vi "探头启用设置.vi"() -> ()   [LabVIEW 2016, in "斯坦道多参数.lvlib"]
uses:
  <vilib>/Utility/miscctls.llb/LVPointTypeDef.ctl
panel:
  in  "藻密度单位":enum16{"cells/mL", "cells/L"}(ring)
  in  "叶绿素a单位":enum16{"μg/L", "mg/L"}(ring)
  in  "关闭":bool
  in  "水温通道":u16(ring)=1 items=["pH", "DO", "浊度", "电导率", "叶绿素a", "藻密度"]
  in  "DO2探头选择":u16(ring)=1 items=["YL型", "MQ型", "NAQ型"]
  in  "DO2启用":bool
  in  "COD探头选择":u16(ring)=1 items=["YL型", "MQ型", "NAQ型"]
  in  "COD启用":bool
  in  "pH":bool
  in  "DO":bool
  in  "Turb":bool
  in  "Cond":bool
  in  "Temp":bool
  in  "叶绿素a启用":bool
  in  "藻密度":bool
  in  "pH探头选择":u16(ring) items=["YL型", "MQ型", "NAQ型"]
  in  "DO探头选择":u16(ring) items=["YL型", "MQ型", "NAQ型"]
  in  "电导率探头选择":u16(ring) items=["YL型", "MQ型", "NAQ型"]
  in  "浊度探头选择":u16(ring) items=["YL型", "MQ型", "NAQ型"]
  in  "叶绿素a探头选择":u16(ring) items=["YL型", "MQ型", "NAQ型"]
  in  "藻密度探头选择":u16(ring) items=["YL型", "MQ型", "NAQ型"]
  in  "ORP启用":bool
  in  "ORP探头选择":u16(ring) items=["YL型", "MQ型", "NAQ型"]
  # "请选择要启用的参数"
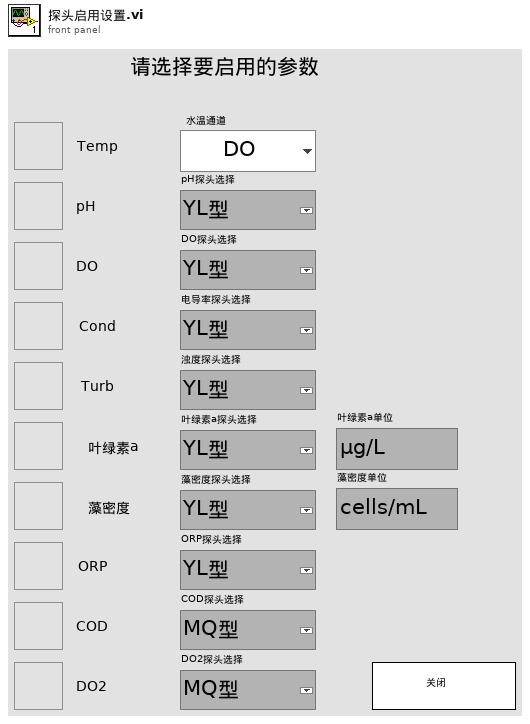
[diagram p1: front panel]
types:
  T1 = typedef "LVPointTypeDef.ctl" = cluster{"Horizontal":i16, "Vertical":i16}
  T2 = cluster{"pH探头选择":u16, "DO探头选择":u16, "电导率探头选择":u16, "浊度探头选择":u16, "叶绿素a探头选择":u16, "蓝绿藻探头选择":u16, "orp探头选择":u16, "COD探头选择":u16, "DO2探头选择":u16}
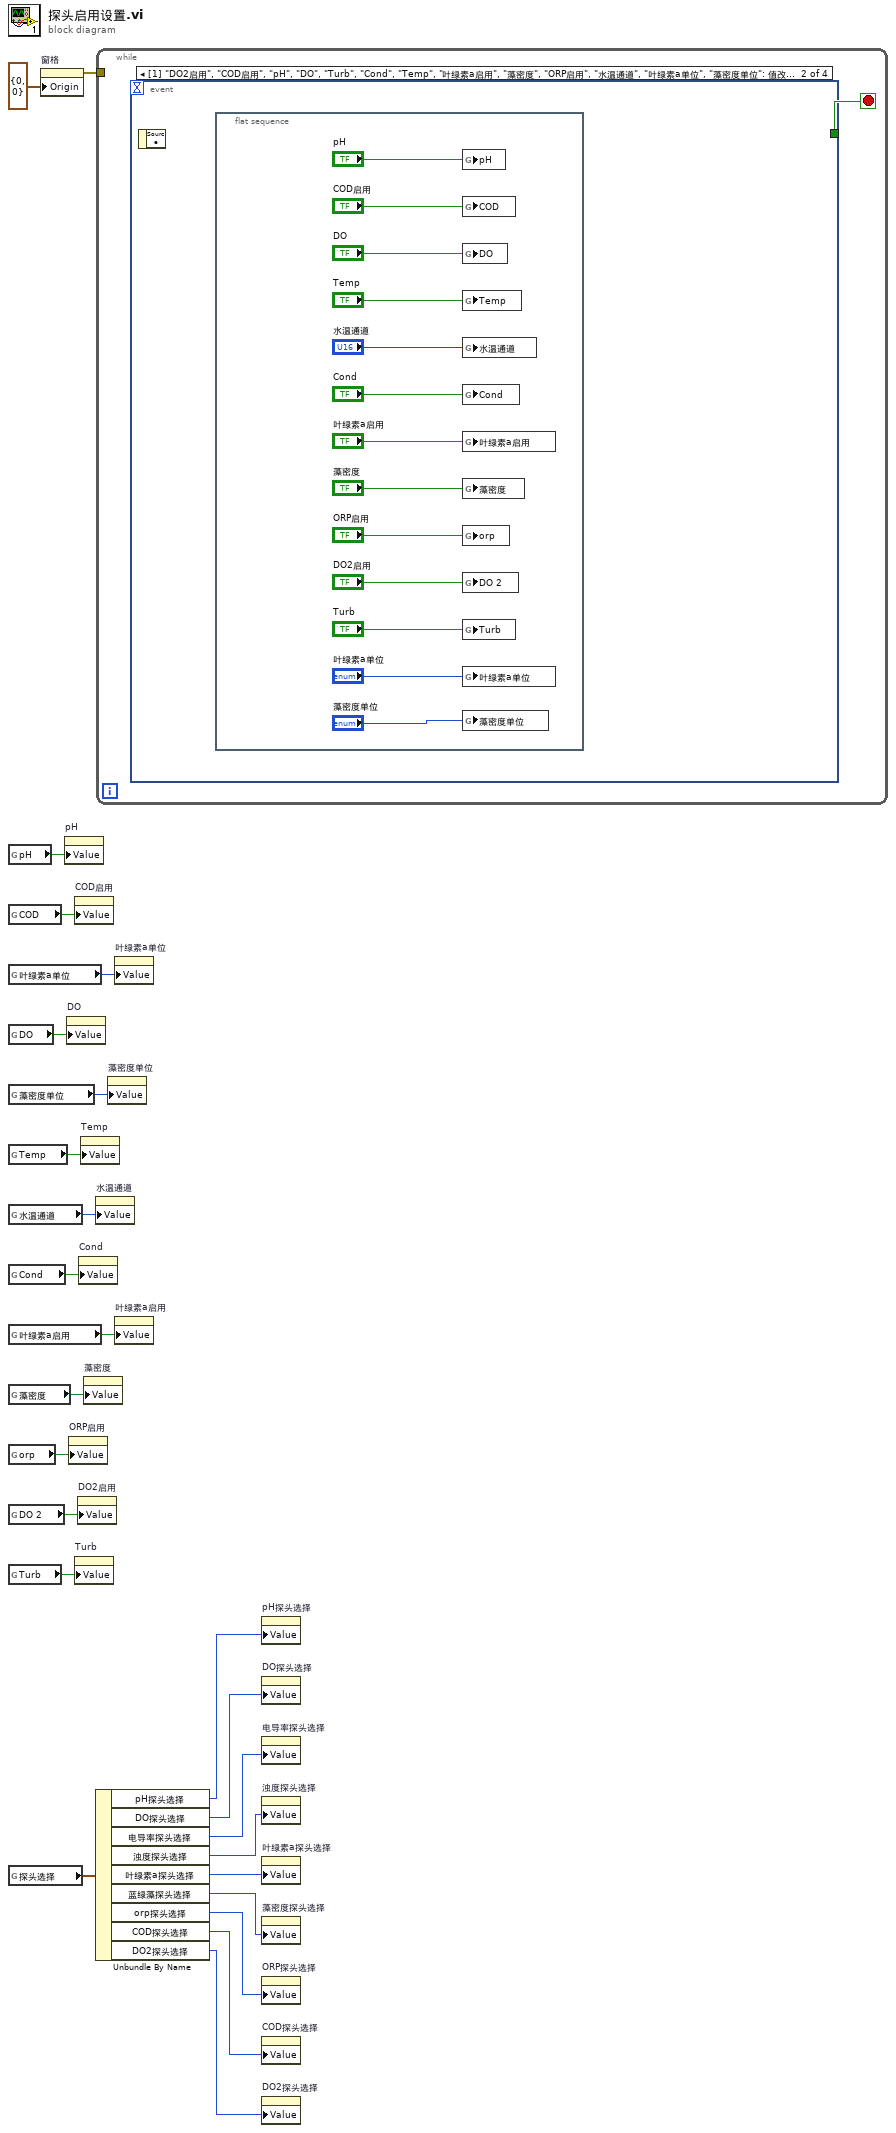
[diagram p0: block diagram]
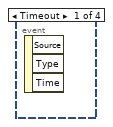
[diagram p2: hidden frame]
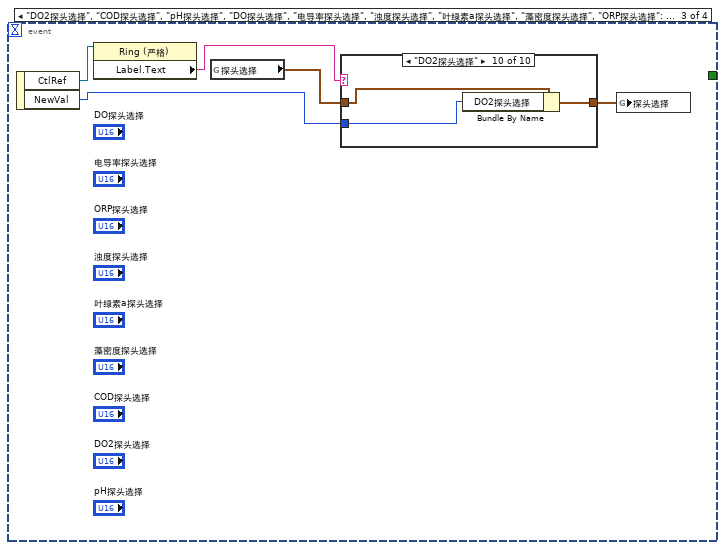
[diagram p3: hidden frame]
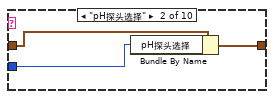
[diagram p5: hidden frame]
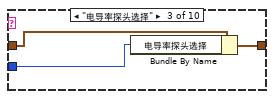
[diagram p6: hidden frame]
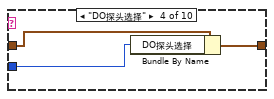
[diagram p7: hidden frame]
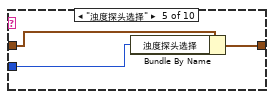
[diagram p8: hidden frame]
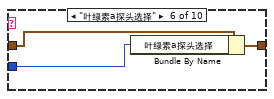
[diagram p9: hidden frame]
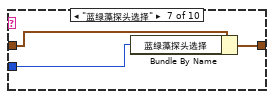
[diagram p10: hidden frame]
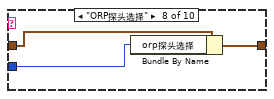
[diagram p11: hidden frame]
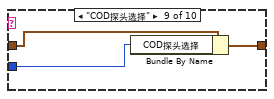
[diagram p12: hidden frame]
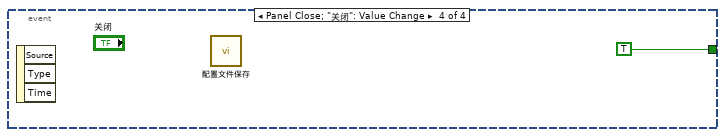
[diagram p13: hidden frame]
diagram:
  n1 = global read "断电保存变量.vi" "pH"() -> (w23:bool)
  n2 = global read "断电保存变量.vi" "COD"() -> (w22:bool)
  n3 = global read "断电保存变量.vi" "叶绿素a单位"() -> (w1:enum16{"μg/L", "mg/L"})
  n4 = global read "断电保存变量.vi" "DO"() -> (w21:bool)
  n5 = global read "断电保存变量.vi" "藻密度单位"() -> (w2:enum16{"cells/mL", "cells/L"})
  n6 = global read "断电保存变量.vi" "Temp"() -> (w20:bool)
  n7 = global read "断电保存变量.vi" "水温通道"() -> (w19:enum16{"pH", "DO", "浊度", "电导率", "叶绿素a", "藻密度"})
  n8 = global read "断电保存变量.vi" "Cond"() -> (w18:bool)
  n9 = global read "断电保存变量.vi" "叶绿素a启用"() -> (w17:bool)
  n10 = global read "断电保存变量.vi" "藻密度"() -> (w16:bool)
  n11 = global read "断电保存变量.vi" "orp"() -> (w15:bool)
  n12 = global read "断电保存变量.vi" "DO 2"() -> (w14:bool)
  n13 = global read "断电保存变量.vi" "Turb"() -> (w13:bool)
  n14 = global read "断电保存变量.vi" "探头选择"() -> (w12:T2)
  n15 = property on="窗格" class="Pane"("Origin"=T1 {"Horizontal"=0, "Vertical"=0} ("原点")) -> (error out=w24:errorcluster)  [unwired: 2 in, 1 out]
  n16 = property on="pH" class="Bool (严格)"("Value"=w23) -> ()  [unwired: 2 in, 2 out]
  n17 = property on="DO" class="Bool (严格)"("Value"=w21) -> ()  [unwired: 2 in, 2 out]
  n18 = property on="ORP启用" class="Bool (严格)"("Value"=w15) -> ()  [unwired: 2 in, 2 out]
  n19 = property on="COD启用" class="Bool (严格)"("Value"=w22) -> ()  [unwired: 2 in, 2 out]
  n20 = property on="Turb" class="Bool (严格)"("Value"=w13) -> ()  [unwired: 2 in, 2 out]
  n21 = property on="DO2启用" class="Bool (严格)"("Value"=w14) -> ()  [unwired: 2 in, 2 out]
  n22 = property on="Cond" class="Bool (严格)"("Value"=w18) -> ()  [unwired: 2 in, 2 out]
  n23 = property on="Temp" class="Bool (严格)"("Value"=w20) -> ()  [unwired: 2 in, 2 out]
  n24 = property on="藻密度" class="Bool (严格)"("Value"=w16) -> ()  [unwired: 2 in, 2 out]
  n25 = property on="水温通道" class="Ring (严格)"("Value"=w19) -> ()  [unwired: 2 in, 2 out]
  n26 = Unbundle By Name(w12) -> ("pH探头选择"=w11:u16, "DO探头选择"=w10:u16, "电导率探头选择"=w9:u16, "浊度探头选择"=w8:u16, "叶绿素a探头选择"=w7:u16, "蓝绿藻探头选择"=w6:u16, "orp探头选择"=w5:u16, "COD探头选择"=w4:u16, "DO2探头选择"=w3:u16)
  n27 = while {
    tunnel: w24 -> [_]
    stop <- w26 stop-if-true
    n28 = event shown="[1] \"DO2启用\", \"COD启用\", \"pH\", \"DO\", \"Turb\", \"Cond\", \"Temp\", \"叶绿素a启用\", \"藻密度\", \"ORP启用\", \"水温通道\", \"叶绿素a单位\", \"藻密度单位\": 值改变" {
      selector: _ -> [_ _ _ _]
      dyn-events: _ -> [_ _ _ _]
      timeout: _ -> [_ _ _ _]
      tunnel: [_ _ _ TRUE] -> w26
      event Timeout {
        n29 = event-data() -> ()  [unwired: 1 in, 3 out]
      }
      event "DO2启用", "COD启用", "pH", "DO", "Turb", "Cond", "Temp", "叶绿素a启用", "藻密度", "ORP启用", "水温通道", "叶绿素a单位", "藻密度单位": Value Change {
        n30 = event-data() -> ()  [unwired: 1 in, 1 out]
        n31 = flat-sequence {
          frame #0 {
            n32 = global write "断电保存变量.vi" "pH"("pH") -> ()
            n33 = global write "断电保存变量.vi" "COD"("COD启用") -> ()
            n34 = global write "断电保存变量.vi" "DO"("DO") -> ()
            n35 = global write "断电保存变量.vi" "Temp"("Temp") -> ()
            n36 = global write "断电保存变量.vi" "水温通道"("水温通道") -> ()
            n37 = global write "断电保存变量.vi" "Cond"("Cond") -> ()
            n38 = global write "断电保存变量.vi" "叶绿素a启用"("叶绿素a启用") -> ()
            n39 = global write "断电保存变量.vi" "藻密度"("藻密度") -> ()
            n40 = global write "断电保存变量.vi" "orp"("ORP启用") -> ()
            n41 = global write "断电保存变量.vi" "DO 2"("DO2启用") -> ()
            n42 = global write "断电保存变量.vi" "Turb"("Turb") -> ()
            n43 = global write "断电保存变量.vi" "叶绿素a单位"("叶绿素a单位") -> ()
            n44 = global write "断电保存变量.vi" "藻密度单位"("藻密度单位") -> ()
          }
        }
      }
      event "DO2探头选择", "COD探头选择", "pH探头选择", "DO探头选择", "电导率探头选择", "浊度探头选择", "叶绿素a探头选择", "藻密度探头选择", "ORP探头选择": Value Change {
        n45 = event-data() -> ("CtlRef"=w41:refnum<vi>, "NewVal"=w40:u16)  [unwired: 1 in]
        n46 = property class="Ring (严格)"(reference=w41) -> ("Label.Text"=w44:string)  [unwired: 1 in, 2 out]
        n47 = global read "断电保存变量.vi" "探头选择"() -> (w43:T2)
        n48 = case shown="\"DO2探头选择\"" w44 {
          tunnel: w43 -> [w45 w48 w51 w54 w57 w60 w63 w66 w69 w72]
          tunnel: [w45 w47 w50 w53 w56 w59 w62 w65 w68 w71] -> w42
          tunnel: w40 -> [_ w46 w49 w52 w55 w58 w61 w64 w67 w70]
          frame Default {
          }
          frame "pH探头选择" {
            n49 = Bundle By Name(cluster=w48, "pH探头选择"=w46) -> (w47:T2)
          }
          frame "电导率探头选择" {
            n50 = Bundle By Name(cluster=w51, "电导率探头选择"=w49) -> (w50:T2)
          }
          frame "DO探头选择" {
            n51 = Bundle By Name(cluster=w54, "DO探头选择"=w52) -> (w53:T2)
          }
          frame "浊度探头选择" {
            n52 = Bundle By Name(cluster=w57, "浊度探头选择"=w55) -> (w56:T2)
          }
          frame "叶绿素a探头选择" {
            n53 = Bundle By Name(cluster=w60, "叶绿素a探头选择"=w58) -> (w59:T2)
          }
          frame "蓝绿藻探头选择" {
            n54 = Bundle By Name(cluster=w63, "蓝绿藻探头选择"=w61) -> (w62:T2)
          }
          frame "ORP探头选择" {
            n55 = Bundle By Name(cluster=w66, "orp探头选择"=w64) -> (w65:T2)
          }
          frame "COD探头选择" {
            n56 = Bundle By Name(cluster=w69, "COD探头选择"=w67) -> (w68:T2)
          }
          frame "DO2探头选择" {
            n57 = Bundle By Name(cluster=w72, "DO2探头选择"=w70) -> (w71:T2)
          }
        }
        n58 = global write "断电保存变量.vi" "探头选择"(w42) -> ()
      }
      event Panel Close; "关闭": Value Change {
        n59 = event-data() -> ()  [unwired: 1 in, 3 out]
        n60 = call "配置文件保存.vi"() -> ()  [unwired: 12 in]
      }
    }
  }
  n61 = property on="藻密度单位" class="Enum (严格)"("Value"=w2) -> ()  [unwired: 2 in, 2 out]
  n62 = property on="叶绿素a单位" class="Enum (严格)"("Value"=w1) -> ()  [unwired: 2 in, 2 out]
  n63 = property on="叶绿素a启用" class="Bool (严格)"("Value"=w17) -> ()  [unwired: 2 in, 2 out]
  n64 = property on="pH探头选择" class="Ring (严格)"("Value"=w11) -> ()  [unwired: 2 in, 2 out]
  n65 = property on="DO探头选择" class="Ring (严格)"("Value"=w10) -> ()  [unwired: 2 in, 2 out]
  n66 = property on="电导率探头选择" class="Ring (严格)"("Value"=w9) -> ()  [unwired: 2 in, 2 out]
  n67 = property on="浊度探头选择" class="Ring (严格)"("Value"=w8) -> ()  [unwired: 2 in, 2 out]
  n68 = property on="叶绿素a探头选择" class="Ring (严格)"("Value"=w7) -> ()  [unwired: 2 in, 2 out]
  n69 = property on="藻密度探头选择" class="Ring (严格)"("Value"=w6) -> ()  [unwired: 2 in, 2 out]
  n70 = property on="ORP探头选择" class="Ring (严格)"("Value"=w5) -> ()  [unwired: 2 in, 2 out]
  n71 = property on="COD探头选择" class="Ring (严格)"("Value"=w4) -> ()  [unwired: 2 in, 2 out]
  n72 = property on="DO2探头选择" class="Ring (严格)"("Value"=w3) -> ()  [unwired: 2 in, 2 out]
